vi "Get Amount of Pyramid Levels.vi"(1 "X Resolution":i32) -> (0 "Pyr Levels":i32)   [LabVIEW 2023]
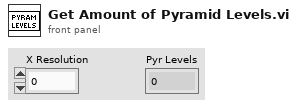
[diagram p1: front panel]
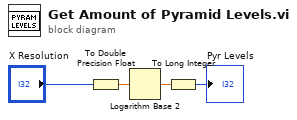
[diagram p0: block diagram]
diagram:
  n1 = To Double Precision Float(number="X Resolution") -> (double precision float=w4:dbl)
  n2 = Logarithm Base 2(1:w4) -> (0:w2:dbl)
  n3 = To Long Integer(number=w2) -> (32bit integer=→"Pyr Levels":i32)
